vi "PH_PSDBWriter.get Instance ID.vi"(1 "PSDB Credentials":T1={"PW"="N/A", "ID"="N/A", "DS"="N/A"}, 2 "Instace Name":string, 3 "Class":string, 4 "Subsystem":string, 5 "error in":errorcluster) -> (17 "instance_id":i32, 19 "error out":errorcluster)   [LabVIEW 2014, in "PH_PSDBWriter.lvlib"]
uses:
  PH_PSDBWriter.lvlib
  PH_Common/Connection/PH_Connection.PSDB Credentials.ctl
  User/Eisenbarth/psdb_lv/PSDB.lvlib
  PH_Common/PH_Common.lvlib
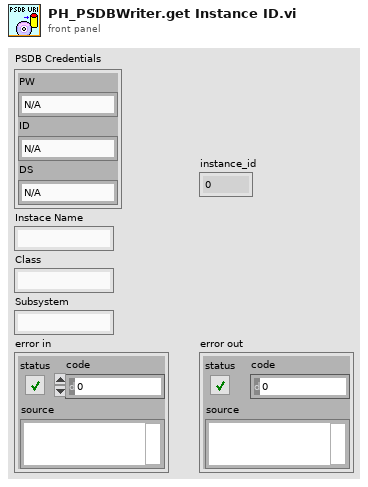
[diagram p1: front panel]
types:
  T1 = typedef "PH_Common.lvlib/PH_Connection.PSDB Credentials.ctl" = cluster{"PW":string, "ID":string, "DS":string}
  T2 = typedef "NI_Database_API.lvlib/Conn ObjectReference.ctl" = refnum<k1>
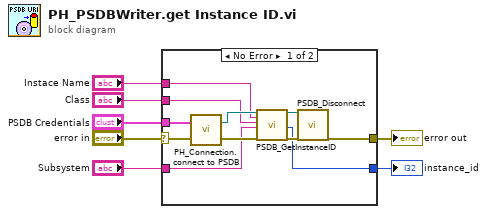
[diagram p0: block diagram]
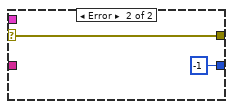
[diagram p2: hidden frame]
diagram:
  n1 = case shown="No Error" "error in" {
    selector: "error in" -> [w9 w20]
    tunnel: [w18 w20] -> w7
    tunnel: [w13 -1 ("instance_id")] -> w6
    tunnel: "Subsystem" -> [w12 _]
    tunnel: "Instace Name" -> [w11 _]
    tunnel: "Class" -> [w10 _]
    tunnel: "PSDB Credentials" -> [w8 _]
    frame No Error {
      n2 = call "PH_Connection.connect to PSDB.vi"("error in"=w9, "PSDB Credentials"=w8) -> ("error out"=w17:errorcluster, "connection reference"=w16:T2)
      n3 = call "PSDB_GetInstanceID.vi"("connection reference"=w16, "Instance"=w11, "Classtype"=w10, "Subsystem"=w12, "error in (no error)"=w17) -> ("connection reference out"=w15:T2, "instance_id"=w13:i32, "error out"=w14:errorcluster)  [unwired: 12 in]
      n4 = call "PSDB_Disconnect.vi"("connection reference"=w15, "error in (no error)"=w14) -> ("error out"=w18:errorcluster)  [unwired: 17 in]
    }
    frame Error {
    }
  }
  "error out" <- w7
  "instance_id" <- w6
